vi "make_unit_set.vi"(7 "unit_set in":variant, 8 "error in (no error)":errorcluster, 10 "symbols []":string[](array[string]), 11 "units []":T1[](array[typedef])) -> (0 "error out":errorcluster, 3 "unit_set out":variant)   [LabVIEW 2015, in "lv-unit-conversion.lvlib"]
uses:
  lv-unit-conversion.lvlib
  _controls/unit_set.ctl
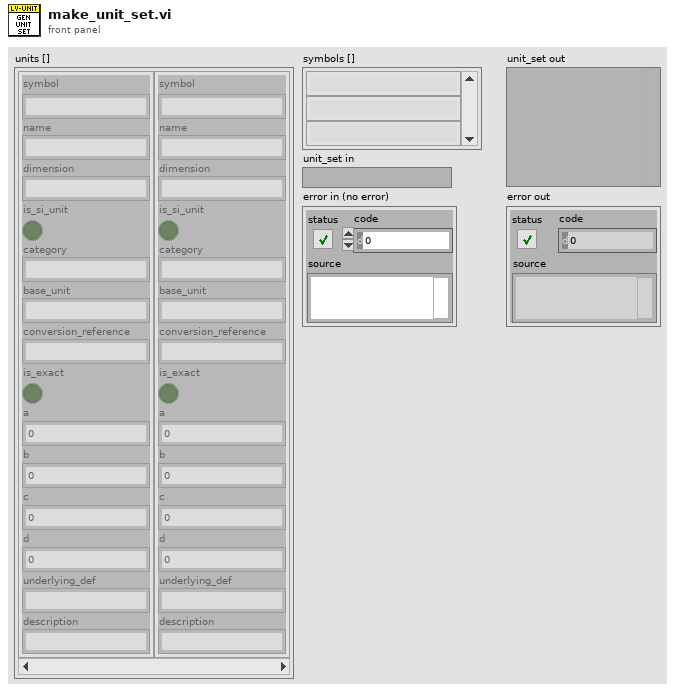
[diagram p1: front panel]
types:
  T1 = typedef "lv-unit-conversion.lvlib/unit_set.ctl" = cluster{"symbol":string, "name":string, "dimension":string, "is_si_unit":bool, "category":string, "base_unit":string, "conversion_reference":string, "is_exact":bool, "a":dbl, "b":dbl, "c":dbl, "d":dbl, "underlying_def":string, "description":string}
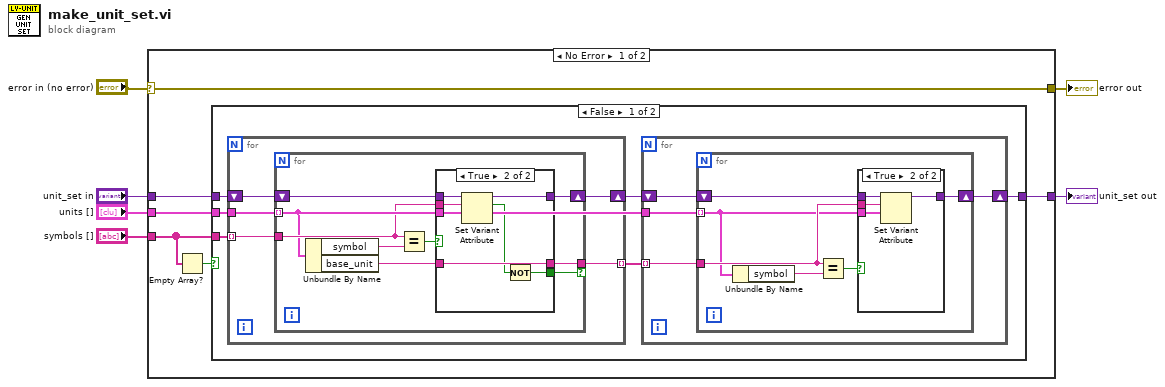
[diagram p0: block diagram]
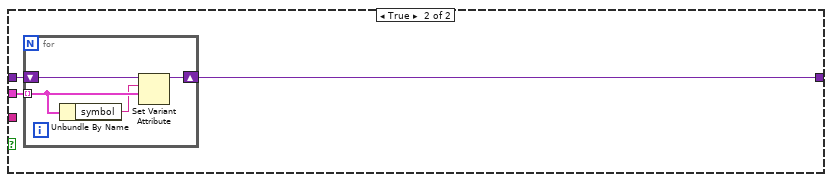
[diagram p4: hidden frame]
diagram:
  n1 = case shown="No Error" "error in (no error)" {
    selector: "error in (no error)" -> [w11 w64]
    tunnel: [w7 w63] -> w6
    tunnel: "units []" -> [w12 _]
    tunnel: "symbols []" -> [w9 _]
    tunnel: "unit_set in" -> [w10 w63]
    tunnel: [w11 w64] -> w1
    frame No Error {
      n2 = Empty Array?(array=w9) -> (empty?=w8:bool)
      n3 = case shown="False" w8 {
        tunnel: w12 -> [w15 w58]
        tunnel: [w13 w57] -> w7
        tunnel: w9 -> [w18 _]
        tunnel: w10 -> [w17 w56]
        frame False {
          n4 = for {
            shift-right: [w37] -> w16
            shift-left: w17 -> [w38]
            tunnel: w18 -> [w35] mode=indexing
            tunnel: w15 -> [w36]
            tunnel: [w34] -> w14 mode=indexing
            n5 = for {
              shift-right: [w46] -> w37
              shift-left: w38 -> [w47]
              tunnel: w36 -> [w42] mode=indexing
              tunnel: w35 -> [w44]
              tunnel: [w40] -> w34 if=w39
              n6 = Unbundle By Name(w42) -> ("symbol"=w45:string, "base_unit"=w41:string)
              n7 = Equal?(x=w44, y=w45) -> (x = y?=w43:bool)
              n8 = case shown="True" w43 {
                tunnel: w47 -> [w48 w55]
                tunnel: [w48 w54] -> w46
                tunnel: w44 -> [_ w53]
                tunnel: w42 -> [_ w52]
                tunnel: w41 -> [_ w51]
                tunnel: [_ w51] -> w40
                tunnel: [_ w49] -> w39
                frame False {
                }
                frame True {
                  n9 = Set Variant Attribute(Variant=w55, name=w53, value=w52) -> (Variant out=w54:variant, replaced=w50:bool)  [unwired: 1 in, 1 out]
                  n10 = Not(x=w50) -> (.not. x?=w49:bool)
                }
              }
            }
          }
          n11 = for {
            shift-right: [w21] -> w13
            shift-left: w16 -> [w22]
            tunnel: w14 -> [w19] mode=indexing
            tunnel: w15 -> [w20]
            n12 = for {
              shift-right: [w27] -> w21
              shift-left: w22 -> [w28]
              tunnel: w20 -> [w23] mode=indexing
              tunnel: w19 -> [w25]
              n13 = Unbundle By Name(w23) -> ("symbol"=w26:string)
              n14 = Equal?(x=w25, y=w26) -> (x = y?=w24:bool)
              n15 = case shown="True" w24 {
                tunnel: w28 -> [w29 w33]
                tunnel: [w29 w32] -> w27
                tunnel: w25 -> [_ w31]
                tunnel: w23 -> [_ w30]
                frame False {
                }
                frame True {
                  n16 = Set Variant Attribute(Variant=w33, name=w31, value=w30) -> (Variant out=w32:variant)  [unwired: 1 in, 2 out]
                }
              }
            }
          }
        }
        frame True {
          n17 = for {
            shift-right: [w61] -> w57
            shift-left: w56 -> [w62]
            tunnel: w58 -> [w60] mode=indexing
            n18 = Unbundle By Name(w60) -> ("symbol"=w59:string)
            n19 = Set Variant Attribute(Variant=w62, name=w59, value=w60) -> (Variant out=w61:variant)  [unwired: 1 in, 2 out]
          }
        }
      }
    }
    frame Error {
    }
  }
  "unit_set out" <- w6
  "error out" <- w1
